vi "Handle Errors.vi"(8 "error in":errorcluster, 11 "eCRDS in":refnum<class "eCRDS.lvclass">) -> (0 "error out":errorcluster, 2 "errors":errorcluster[](array[cluster]), 3 "eCRDS out":refnum<class "eCRDS.lvclass">)   [LabVIEW 2014, in "eCRDS Library.lvlib" / "eCRDS.lvclass"]
uses:
  eCRDS.lvclass
  eCRDS.lvclass/eCRDS.ctl
  reusable/CRDS/Main/CRDS.lvclass
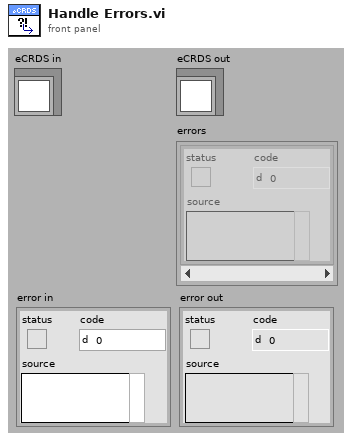
[diagram p1: front panel]
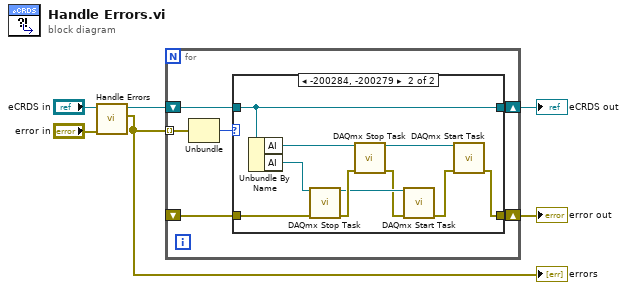
[diagram p0: block diagram]
diagram:
  n1 = call-parent "Handle Errors.vi"("error in"="error in", "Instrument in"="eCRDS in") -> ("errors"=w2:errorcluster[], "Instrument out"=w4:refnum<class "eCRDS.lvclass">)  [unwired: 7 in, 1 out]
  "errors" <- w2
  n2 = for {
    tunnel: w2 -> [w12] mode=indexing
    shift-right: [w9] -> w3
    shift-left: w4 -> [w10]
    shift-right: [w8] -> w1
    shift-left: _ -> [w7]
    n3 = Unbundle(w12) -> ("code"=w11:i32)  [unwired: 2 out]
    n4 = case shown="-200284, -200279" w11 {
      tunnel: w10 -> [w14 w17]
      tunnel: [w14 w17] -> w9
      tunnel: [w13 w16] -> w8
      tunnel: w7 -> [w13 w15]
      frame 0, Default {
      }
      frame -200284, -200279 {
        n5 = Unbundle By Name(w17) -> ("AI"=w24:refnum<k21>, "AI"=w23:refnum<k21>)
        n6 = call <vilib>:"DAQmx Stop Task.vi"("task/channels in"=w23, "error in"=w15) -> ("task out"=w21:refnum<k21>, "error out"=w22:errorcluster)  [unwired: 12 in]
        n7 = call <vilib>:"DAQmx Stop Task.vi"("task/channels in"=w24, "error in"=w22) -> ("task out"=w18:refnum<k21>, "error out"=w20:errorcluster)  [unwired: 12 in]
        n8 = call <vilib>:"DAQmx Start Task.vi"("task/channels in"=w21, "error in"=w20) -> ("error out"=w19:errorcluster)  [unwired: 12 in, 1 out]
        n9 = call <vilib>:"DAQmx Start Task.vi"("task/channels in"=w18, "error in"=w19) -> ("error out"=w16:errorcluster)  [unwired: 12 in, 1 out]
      }
    }
  }
  "error out" <- w1
  "eCRDS out" <- w3
